vi "ep_Check Duplicated Physical Channel Index.vi"(8 "error in (no error)":errorcluster, 9 "number of channels":i32, 10 "current channels":T1[](array[typedef]) {"physical channels"."channel phase" items=["Phase A (L1)", "Phase B (L2)", "Phase C (L3)", "Phase N (Neutral)"]}, 11 "voltage channels":T1[](array[typedef]) {"physical channels"."channel phase" items=["Phase A (L1)", "Phase B (L2)", "Phase C (L3)", "Phase N (Neutral)"]}) -> (0 "error out":errorcluster)   [LabVIEW 2014, in "NI_EP_Power Quality.lvlib"]
uses:
  <vilib>/addons/Electrical Power/PQ/NI_EP_Power Quality.lvlib
  <vilib>/addons/Electrical Power/PQ/Common/Controls/ep_Channels Config.ctl
  <vilib>/addons/Electrical Power/PQ/Common/Controls/ep_Channel Phase.ctl
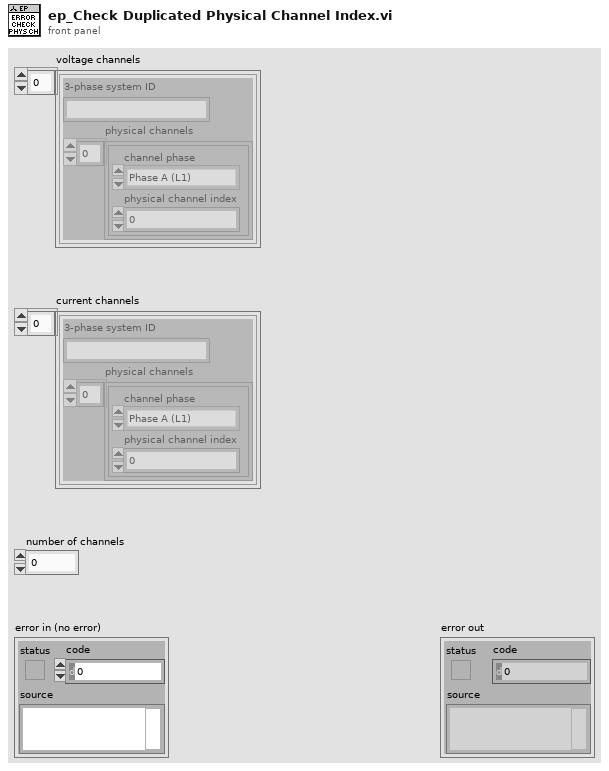
[diagram p1: front panel]
types:
  T1 = typedef "NI_EP_Power Quality.lvlib/ep_Channels Config.ctl" = cluster{"3-phase system ID":string, "physical channels":cluster{"channel phase":T2, "physical channel index":u16}[]}
  T2 = typedef "NI_EP_Power Quality.lvlib/ep_Channel Phase.ctl" = u16
  T3 = cluster{"channel phase":T2, "physical channel index":u16}[]
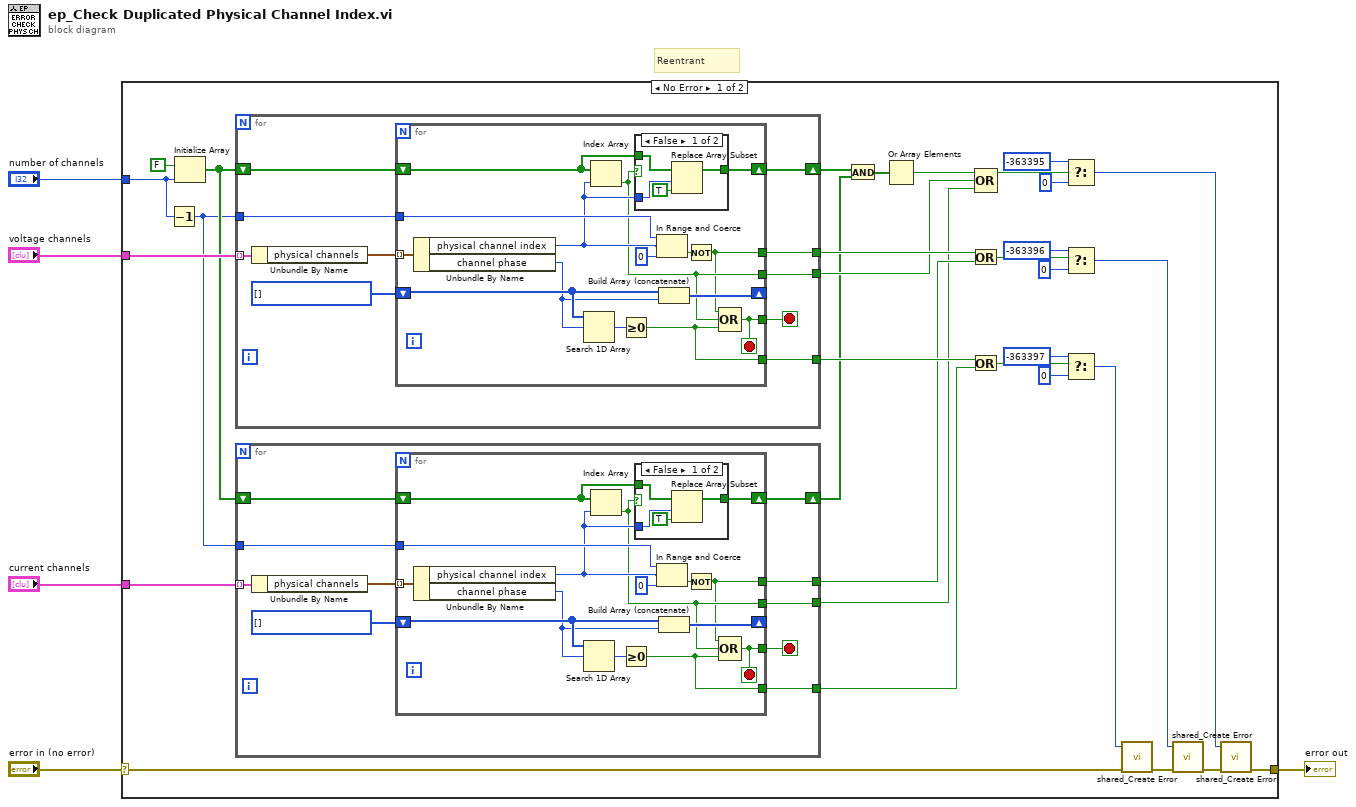
[diagram p0: block diagram]
diagram:
  # "Reentrant"
  n1 = case shown="No Error" "error in (no error)" {
    selector: "error in (no error)" -> [w16 w98]
    tunnel: "voltage channels" -> [w37 _]
    tunnel: "current channels" -> [w10 _]
    tunnel: [w35 w98] -> w4
    tunnel: "number of channels" -> [w23 _]
    frame No Error {
      n2 = Decrement(x=w23) -> (x-1=w11:i32)
      n3 = Initialize Array(FALSE, w23) -> (w12:bool[])
      n4 = for {
        tunnel: w37 -> [w77] mode=indexing
        shift-right: [w75] -> w33
        shift-left: w12 -> [w76]
        tunnel: w11 -> [w74]
        tunnel: [w71] -> w14
        tunnel: [w70] -> w15
        tunnel: [w69] -> w13
        stop <- w72 stop-if-true
        w73 = T2[] [] items=["Phase A (L1)", "Phase B (L2)", "Phase C (L3)", "Phase N (Neutral)"]
        n5 = Unbundle By Name(w77) -> ("physical channels"=w68:T3)
        n6 = for {
          tunnel: w68 -> [w92] mode=indexing
          shift-right: [w91] -> w75
          shift-left: w76 -> [w80]
          tunnel: w74 -> [w89]
          shift-right: [w85] -> _
          shift-left: w73 -> [w88]
          tunnel: [w84] -> w72
          tunnel: [w78] -> w71
          tunnel: [w82] -> w70
          tunnel: [w79] -> w69
          stop <- w84 stop-if-true
          n7 = Unbundle By Name(w92) -> ("physical channel index"=w81:u16, "channel phase"=w86:T2)
          n8 = Search 1D Array(1D array=w88, element=w86) -> (index of element=w87:i32)  [unwired: 1 in]
          n9 = Index Array(array=w80, index=w81) -> (element=w79:bool)
          n10 = Greater Or Equal To 0?(x=w87) -> (x >= 0?=w82:bool)
          n11 = case shown="False" w79 {
            tunnel: [w96 w97] -> w91
            tunnel: w81 -> [w94 _]
            tunnel: w80 -> [w93 w97]
            frame False {
              n12 = Replace Array Subset(array=w93, new element=TRUE ("new element/subarray"), index=w94) -> (w96:bool[])
            }
            frame True {
            }
          }
          n13 = In Range and Coerce(upper limit=w89, x=w81, lower limit=0) -> (In Range?=w83:bool)  [unwired: 1 out]
          n14 = Build Array (concatenate)(w88, w86) -> (w85:T2[])
          n15 = Not(x=w83) -> (.not. x?=w78:bool)
          n16 = Compound Arithmetic op=OR(w78, w79, w82) -> (w84:bool)
        }
      }
      n17 = for {
        tunnel: w10 -> [w47] mode=indexing
        shift-right: [w45] -> w9
        shift-left: w12 -> [w46]
        tunnel: w11 -> [w44]
        tunnel: [w41] -> w8
        tunnel: [w40] -> w6
        tunnel: [w39] -> w7
        stop <- w42 stop-if-true
        w43 = T2[] [] items=["Phase A (L1)", "Phase B (L2)", "Phase C (L3)", "Phase N (Neutral)"]
        n18 = Unbundle By Name(w47) -> ("physical channels"=w38:T3)
        n19 = for {
          tunnel: w38 -> [w62] mode=indexing
          shift-right: [w61] -> w45
          shift-left: w46 -> [w50]
          tunnel: w44 -> [w59]
          shift-right: [w55] -> _
          shift-left: w43 -> [w58]
          tunnel: [w54] -> w42
          tunnel: [w48] -> w41
          tunnel: [w52] -> w40
          tunnel: [w49] -> w39
          stop <- w54 stop-if-true
          n20 = Unbundle By Name(w62) -> ("physical channel index"=w51:u16, "channel phase"=w56:T2)
          n21 = Search 1D Array(1D array=w58, element=w56) -> (index of element=w57:i32)  [unwired: 1 in]
          n22 = Index Array(array=w50, index=w51) -> (element=w49:bool)
          n23 = Greater Or Equal To 0?(x=w57) -> (x >= 0?=w52:bool)
          n24 = case shown="False" w49 {
            tunnel: [w66 w67] -> w61
            tunnel: w51 -> [w64 _]
            tunnel: w50 -> [w63 w67]
            frame False {
              n25 = Replace Array Subset(array=w63, new element=TRUE ("new element/subarray"), index=w64) -> (w66:bool[])
            }
            frame True {
            }
          }
          n26 = In Range and Coerce(upper limit=w59, x=w51, lower limit=0) -> (In Range?=w53:bool)  [unwired: 1 out]
          n27 = Build Array (concatenate)(w58, w56) -> (w55:T2[])
          n28 = Not(x=w53) -> (.not. x?=w48:bool)
          n29 = Compound Arithmetic op=OR(w48, w49, w52) -> (w54:bool)
        }
      }
      n30 = And(x=w33, y=w9) -> (x .and. y?=w32:bool[])
      n31 = Or Array Elements(Boolean array=w32) -> (logical OR=w26:bool)
      n32 = Or(x=w14, y=w8) -> (x .or. y?=w31:bool)
      n33 = Or(x=w15, y=w6) -> (x .or. y?=w22:bool)
      n34 = Compound Arithmetic op=OR(w26, w13, w7) -> (w17:bool)
      n35 = Select(t=-363395, s=w17, f=0) -> (s? t:f=w36:i32)
      n36 = Select(t=-363396, s=w31, f=0) -> (s? t:f=w29:i32)
      n37 = Select(t=-363397, s=w22, f=0) -> (s? t:f=w21:i32)
      n38 = call <vilib>:"shared_Create Error.vi"("error in (no error)"=w16, "error code (0)"=w21) -> ("error out"=w18:errorcluster)  [unwired: 9 in]
      n39 = call <vilib>:"shared_Create Error.vi"("error in (no error)"=w18, "error code (0)"=w29) -> ("error out"=w30:errorcluster)  [unwired: 9 in]
      n40 = call <vilib>:"shared_Create Error.vi"("error in (no error)"=w30, "error code (0)"=w36) -> ("error out"=w35:errorcluster)  [unwired: 9 in]
    }
    frame Error {
    }
  }
  "error out" <- w4
